vi "Handle Errors.vi"(8 "error in (no error)":errorcluster) -> (0 "error out":errorcluster)   [LabVIEW 2020, in "Process.lvclass"]
uses:
  Process.lvclass
  Process.lvclass/Process.ctl
  <vilib>/Utility/sysdir.llb/System Directory Type.ctl
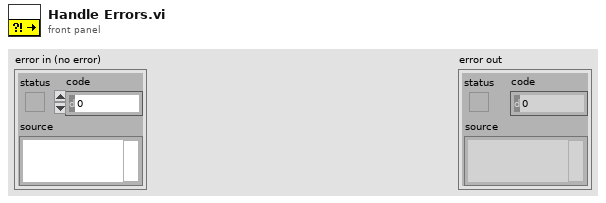
[diagram p1: front panel]
types:
  T1 = enum16{"open", "replace", "create", "open or create", "replace or create", "replace or create with confirmation"}
  T2 = typedef "System Directory Type.ctl" = i32
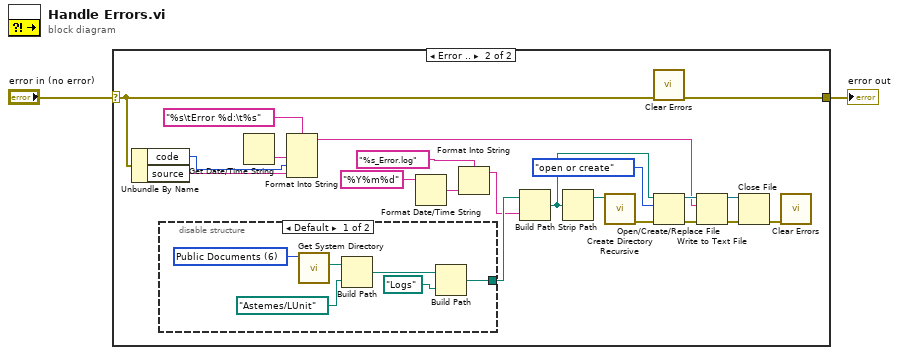
[diagram p0: block diagram]
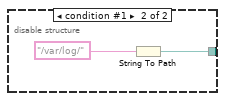
[diagram p3: hidden frame]
diagram:
  n1 = case shown="Error .." "error in (no error)" {
    selector: "error in (no error)" -> [w3 w23]
    tunnel: [w3 w24] -> w1
    frame No Error {
    }
    frame Error {
      n2 = Unbundle By Name(w23) -> ("code"=w7:i32, "source"=w6:string)
      n3 = disable-structure shown="Default" {
        disable-tunnel: [w30 w31] -> w16
        frame condition #0 (active) {
          w25 = T2 6 items=["User Home"=0, "User Desktop"=1, "User Documents"=2, "User Application Data"=3, "User Preferences"=4, "User Temporary"=5, "Public Documents"=6, "Public Application Data"=7, "Public Preferences"=8, "Public Cache"=13, "System Core Libraries"=9, "System Installed Libraries"=10, "Application Files"=11, "Boot Volume Root"=12] ("system directory type")
          n4 = call <vilib>:"Get System Directory.vi"("system directory type"=w25) -> ("system directory"=w27:path)  [unwired: 10 in]
          n5 = Build Path(base path=w27, name or relative path=path "Astemes/LUnit") -> (appended path=w28:path)
          n6 = Build Path(base path=w28, name or relative path=path "Logs") -> (appended path=w30:path)
        }
        frame condition #1 {
          n7 = String To Path(string="/var/log/") -> (path=w31:path)
        }
      }
      n8 = Get Date/Time String() -> (time string=w5:string)  [unwired: 3 in, 1 out]
      n9 = Format Into String(format string="%s\tError %d:\t%s", w5, w7, w6) -> (resulting string=w4:string)  [unwired: 2 in, 1 out]
      n10 = Format Date/Time String(time format string (%c)="%Y%m%d") -> (date/time string=w22:string)  [unwired: 2 in]
      n11 = Format Into String(format string="%s_Error.log", w22) -> (resulting string=w15:string)  [unwired: 2 in, 1 out]
      n12 = Build Path(base path=w16, name or relative path=w15) -> (appended path=w14:path)
      n13 = Strip Path(path=w14) -> (stripped path=w19:path)  [unwired: 1 out]
      n14 = call <vilib>:"Create Directory Recursive.vi"("directory"=w19) -> ("error out"=w20:errorcluster)  [unwired: 4 in, 2 out]
      n15 = call <vilib>:"Clear Errors.vi"("error in (no error)"=w23) -> ("error out"=w24:errorcluster)  [unwired: 5 in, 1 out]
      n16 = Open/Create/Replace File(file path (use dialog)=w14, error in=w20, operation (0:open)=T1."open or create") -> (refnum out=w13:refnum<file>, error out=w12:errorcluster)  [unwired: 3 in, 1 out]
      n17 = Write to Text File(file (use dialog)=w13, text=w4, error in=w12) -> (refnum out=w11:refnum<file>, error out=w10:errorcluster)  [unwired: 1 in, 1 out]
      n18 = Close File(refnum=w11, error in=w10) -> (error out=w9:errorcluster)  [unwired: 1 out]
      n19 = call <vilib>:"Clear Errors.vi"("error in (no error)"=w9) -> ()  [unwired: 5 in, 2 out]
    }
  }
  "error out" <- w1
